vi "Write Buffer to Log.vi"(8 "error in":errorcluster) -> (0 "error out":errorcluster)   [LabVIEW 2017, in "Huskie Swerve.lvlib"]
uses:
  Huskie Swerve.lvlib
  Huskie Board.ctl
  Refname to String (Huskie Board).vi
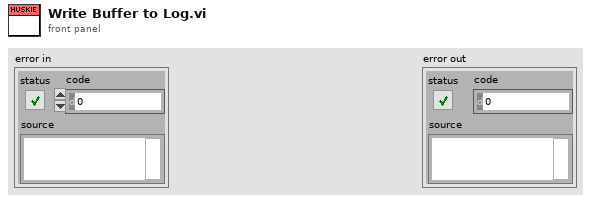
[diagram p1: front panel]
types:
  T1 = typedef "Huskie Swerve.lvlib/Huskie Board.ctl" = enum16{"Huskie Board", "Log Queue", ""}
  T2 = typedef "WPI_SerialPortRef.ctl" = cluster{"DevStatus":errorcluster, "Serial Port Name":refnum<visa-resource-name>}
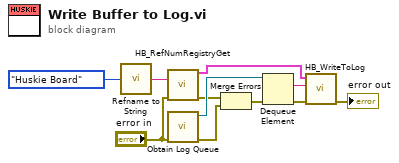
[diagram p0: block diagram]
diagram:
  n1 = call-poly "Refname to String.vi"("Enum"=Huskie_Board."Huskie Board") -> ("resulting string"=w10:string)
  n2 = call <vilib>:"HB_RefNumRegistryGet.vi"("refnum name"=w10, "error in (no error)"="error in") -> ("HBDevRef"=w9:T2, "error out"=w4:errorcluster)  [unwired: 12 in]
  n3 = call "Obtain Log Queue.vi"("error in"="error in") -> ("error out"=w3:errorcluster, "queue out"=w7:refnum<queue>)  [unwired: 9 in]
  n4 = Merge Errors(w4, w3) -> (w5:errorcluster)
  n5 = Dequeue Element(queue=w7, error in (no error)=w5) -> (element=w6:string, error out=w2:errorcluster)  [unwired: 1 in, 2 out]
  n6 = call <vilib>:"HB_WriteToLog.vi"("error in (no error)"=w2, "Log string"=w6, "HBDevRef"=w9) -> ("error out"=→"error out":errorcluster)  [unwired: 7 in, 1 out]
